vi "oldVisionToGame.vi"(6 "Team/ Side":u16[](array[numeric]), 8 "error in (no error)":errorcluster, 10 "IA State":T1={"our_robots"=[], "enemy_robots"=[], "balls"=[], "geometry"={"line_width"=0, "field_length"=0, "field_width"=0, "boundary_width"=0, "referee_width"=0, "goal_width"=0, "goal_depth"=0, "goal_wall_width"=0, "center_circle_radius"=0, "defense_radius"=0, "defense_stretch"=0, "free_kick_from_defense_dist"=0, "penalty_spot_from_field_line_dist"=0, "penalty_line_from_spot_dist"=0}, "IA Judge"={"stage"="", "command"="", "our_goalie_id"=0.0, "enemy_goalie_id"=0.0, "command enum"=enum."Halt", "Time"=enum."Azul"}, "Received Timestamp"=timestamp(0 s since 1904-01-01), "Events"={"Touch"=FALSE, "Ball out"=FALSE, "id touch"=0.0, "Ball out of \nVision"=FALSE, "Ball inside \nGoalie area"=FALSE, "Robot not responding"=FALSE, "Robots responding status"=[1.0, 1.0, 1.0, 1.0, 1.0, 1.0], "Enemy Ball \nPossession"=FALSE, "Pass State"=FALSE, "id end of pass"=0.0, "Kick"=FALSE, "Id ini Possession"=0.0, "Ball Possesion"=FALSE, "Id Possesion"=0.0, "Direct Kick"=FALSE, "2nd Strk Ativo"=FALSE}}, 11 "Game in":refnum<class "Game.lvclass">) -> (0 "error out":errorcluster, 3 "Game out":refnum<class "Game.lvclass">)   [LabVIEW 2018, in "Game.lvclass"]
uses:
  Game.lvclass
  Vision_class/Old vision/Controls/AI Input.ctl
  Vision_class/Old vision/Controls/AI Robot.ctl
  Vision_class/Old vision/Controls/Functions Enum.ctl
  Vision_class/Old vision/Controls/AttackerStates.ctl
  Vision_class/Old vision/Controls/PathDests.ctl
  Vision_class/Old vision/Controls/PathDest.ctl
  Vision_class/Old vision/Controls/AI Ball.ctl
  Vision_class/Old vision/Controls/Field Size.ctl
  Vision_class/Old vision/Controls/AI Judge.ctl
  Vision_class/Old vision/Controls/Command Enum.ctl
  Vision_class/Old vision/Controls/Events.ctl
  Game.lvclass/Game.ctl
  Write FieldRef.vi
  Write AllyRef.vi
  Write EnemyRef.vi
  Write BallRef.vi
  Read FieldRef.vi
  Read AllyRef.vi
  Read EnemyRef.vi
  Read BallRef.vi
  Field_class/Field.lvclass
  Ally_class/Ally.lvclass
  Enemy_class/Enemy.lvclass
  Ball_class/Ball.lvclass
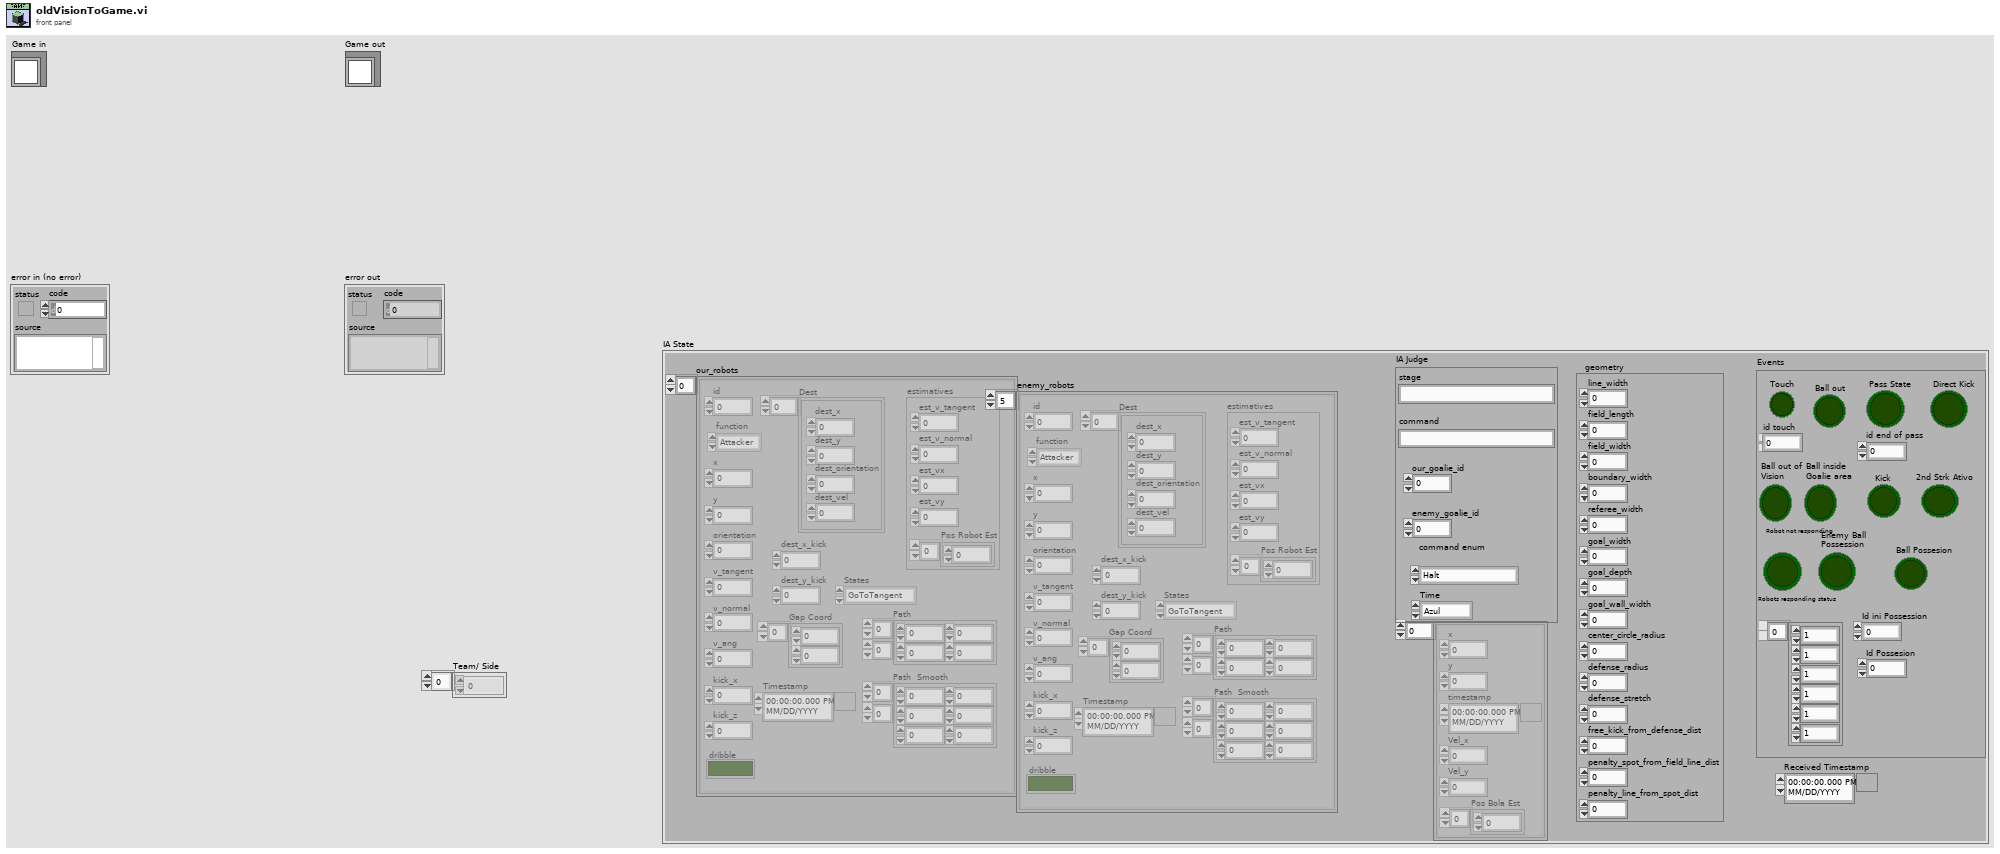
[diagram p1: front panel]
types:
  T1 = typedef "AI Input.ctl" = cluster{"our_robots":T2[], "enemy_robots":T2[], "balls":T7[], "geometry":T8, "IA Judge":T9, "Received Timestamp":timestamp, "Events":T11}
  T2 = typedef "AI Robot.ctl" = cluster{"id":u32, "function":T3, "x":dbl, "y":dbl, "orientation":dbl, "v_tangent":dbl, "v_normal":dbl, "v_ang":dbl, "kick_x":dbl, "kick_z":dbl, "dribble":bool, "Timestamp":timestamp, "estimatives":cluster{"est_v_tangent":dbl, "est_v_normal":dbl, "est_vx":dbl, "est_vy":dbl, "Pos Robot Est":dbl[]}, "dest_x_kick":dbl, "dest_y_kick":dbl, "Gap Coord":dbl[], "States":T4, "Path ":dbl[][], "Path  Smooth":dbl[][], "Dest":T5}
  T3 = typedef "Functions Enum.ctl" = enum16{"2nd Striker", "Attacker", "Goalie", "Defender", "Striker", "Goto 0", "Dummy", "Kicker", "ZigZag 0", "ZigZag 1", "ZigZag 2", "ZigZag 3", "ZigZag 4", "ZigZag 5", "ZigZag 6", "ZigZag 7", "ZigZag 8", ""}
  T4 = typedef "AttackerStates.ctl" = enum16{"Pass", "GoToTangent", "BallGetting", "GoToKick", ""}
  T5 = typedef "PathDests.ctl" = T6[]
  T6 = typedef "PathDest.ctl" = cluster{"dest_x":dbl, "dest_y":dbl, "dest_orientation":dbl, "dest_vel":dbl}
  T7 = typedef "AI Ball.ctl" = cluster{"x":dbl, "y":dbl, "timestamp":timestamp, "Vel_x":dbl, "Vel_y":dbl, "Pos Bola Est":dbl[]}
  T8 = typedef "Field Size.ctl" = cluster{"line_width":u32, "field_length":u32, "field_width":u32, "boundary_width":u32, "referee_width":u32, "goal_width":u32, "goal_depth":u32, "goal_wall_width":u32, "center_circle_radius":u32, "defense_radius":u32, "defense_stretch":u32, "free_kick_from_defense_dist":u32, "penalty_spot_from_field_line_dist":u32, "penalty_line_from_spot_dist":u32}
  T9 = typedef "AI Judge.ctl" = cluster{"stage":string, "command":string, "our_goalie_id":dbl, "enemy_goalie_id":dbl, "command enum":T10, "Time":enum16{"Azul", "Amarelo"}}
  T10 = typedef "Command Enum.ctl" = enum16{"Halt", "Stop", "Force Start", "PKA Normal Start", "Prepare Kickoff Ally", "PKE Normal Start", "Prepare Kickoff Enemy", "Prepare Penalty Ally", "PPA Normal Start", "Prepare Penalty Enemy", "PPE Normal Start", "Direct Free Enemy", "Direct Free Ally", "Indirect Free Enemy", "Indirect Free Ally", "Timeout Enemy", "Timeout Ally", "Goal Enemy", "Goal Ally", "Ball Placement Enemy", "Ball Placement Ally", "Normal Half Time", "Extra Time Break", "Extra Half Time", "None", "Post Game"}
  T11 = typedef "Events.ctl" = cluster{"Touch":bool, "Ball out":bool, "id touch":dbl, "Ball out of \nVision":bool, "Ball inside \nGoalie area":bool, "Robot not responding":bool, "Robots responding status":dbl[], "Enemy Ball \nPossession":bool, "Pass State":bool, "id end of pass":dbl, "Kick":bool, "Id ini Possession":dbl, "Ball Possesion":bool, "Id Possesion":dbl, "Direct Kick":bool, "2nd Strk Ativo":bool}
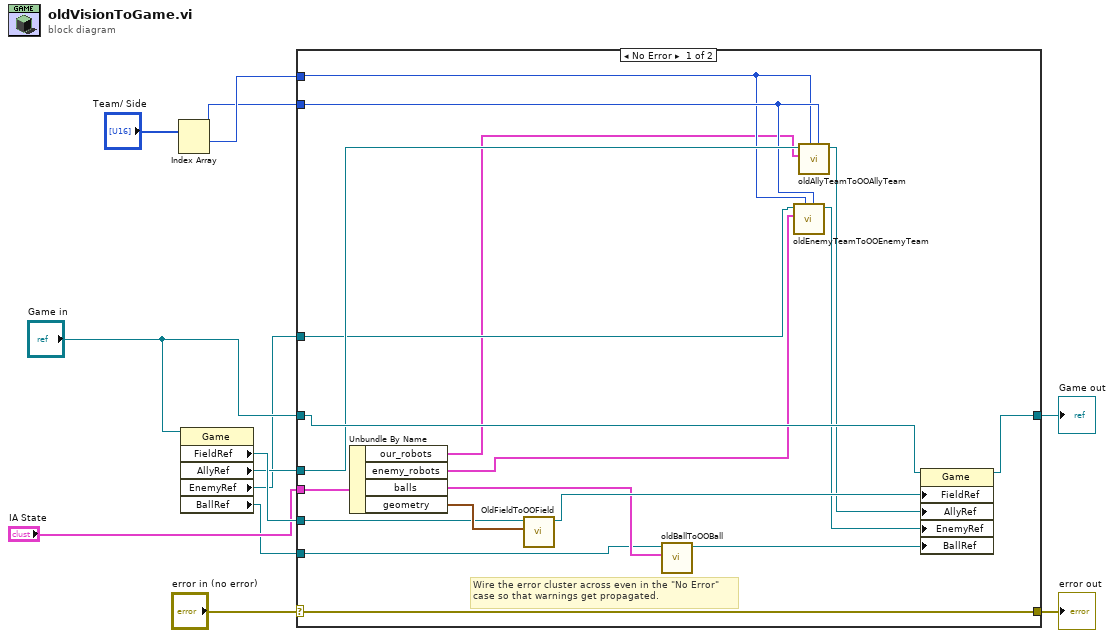
[diagram p0: block diagram]
diagram:
  n1 = Index Array(array="Team/ Side") -> (element #1=w4:u16, element #2=w3:u16)  [unwired: 2 in]
  n2 = property class="Game"(reference="Game in") -> ("FieldRef"=w8:refnum<class "Field.lvclass">, "AllyRef"=w7:refnum<class "Ally.lvclass">, "EnemyRef"=w6:refnum<class "Enemy.lvclass">, "BallRef"=w1:refnum<class "Ball.lvclass">)  [unwired: 1 in, 2 out]
  n3 = case shown="No Error" "error in (no error)" {
    selector: "error in (no error)" -> [w30 w32]
    tunnel: [w30 w32] -> w11
    tunnel: [w25 w31] -> w10
    tunnel: "Game in" -> [w24 w31]
    tunnel: "IA State" -> [w29 _]
    tunnel: w8 -> [w27 _]
    tunnel: w3 -> [w18 _]
    tunnel: w7 -> [w22 _]
    tunnel: w6 -> [w21 _]
    tunnel: w4 -> [w17 _]
    tunnel: w1 -> [w13 _]
    frame No Error {
      # "Wire the error cluster across even in the \"No Error\"\ncase so that warnings get propagated."
      n4 = Unbundle By Name(w29) -> ("our_robots"=w14:T2[], "enemy_robots"=w16:T2[], "balls"=w15:T7[], "geometry"=w28:T8)
      n5 = call "OldFieldToOOField.vi"("geometry"=w28, "Field in"=w27) -> ("Field out"=w26:refnum<class "Field.lvclass">)  [unwired: 8 in, 1 out]
      n6 = call "oldBallToOOBall.vi"("balls"=w15, "Ball in"=w13) -> ("Ball out"=w19:refnum<class "Ball.lvclass">)  [unwired: 8 in, 1 out]
      n7 = call "oldEnemyTeamToOOEnemyTeam.vi"("Side"=w18, "Team"=w17, "enemy_robots"=w16, "Enemy in"=w21) -> ("Enemy out"=w20:refnum<class "Enemy.lvclass">)  [unwired: 6 in, 1 out]
      n8 = call "oldAllyTeamToOOAllyTeam.vi"("Side"=w18, "Team"=w17, "our_robots"=w14, "Ally in"=w22) -> ("Ally out"=w23:refnum<class "Ally.lvclass">)  [unwired: 6 in, 1 out]
      n9 = property class="Game"(reference=w24, "FieldRef"=w26, "AllyRef"=w23, "EnemyRef"=w20, "BallRef"=w19) -> (reference out=w25:refnum<class "Game.lvclass">)  [unwired: 1 in, 1 out]
    }
    frame Error {
    }
  }
  "error out" <- w11
  "Game out" <- w10
